vi "Is Running.vi"(8 "error in (no error)":errorcluster, 11 "SB App in":refnum<class "SB App.lvclass">) -> (0 "error out":errorcluster, 2 "Running":bool, 3 "SB App out":refnum<class "SB App.lvclass">)   [LabVIEW 2020, in "SB App.lvlib" / "SB App.lvclass"]
uses:
  SB App.lvclass
  SB App.lvclass/SB App.ctl
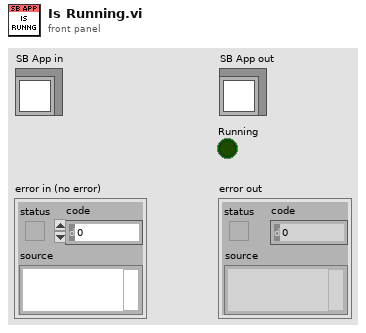
[diagram p1: front panel]
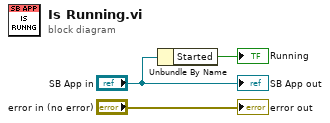
[diagram p0: block diagram]
diagram:
  n1 = Unbundle By Name("SB App in") -> ("Started"=→"Running":bool)
  "error out" <- "error in (no error)"
  "SB App out" <- "SB App in"
